vi "Wrapper Fulfill Future.vi"(8 "error in (no error)":errorcluster, 10 "Variant":variant, 11 "Promise in":refnum<class "Promise.lvclass">) -> (0 "error out":errorcluster)   [LabVIEW 2017, in "Promise Future.lvlib" / "Promise.lvclass"]
uses:
  Promise.lvclass
  Promise.lvclass/Promise.ctl
  Future/Future.lvclass
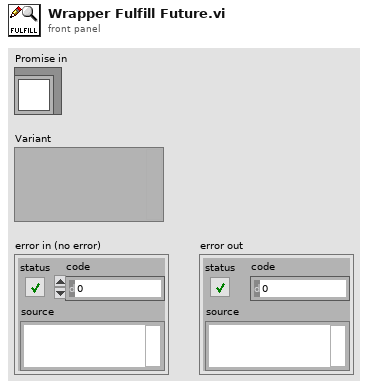
[diagram p1: front panel]
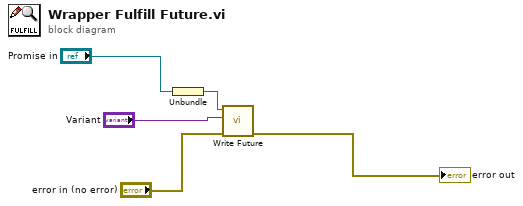
[diagram p0: block diagram]
diagram:
  n1 = Unbundle("Promise in") -> (w1:refnum<class "Future.lvclass">)
  n2 = call "Write Future.vi"("error in (no error)"="error in (no error)", "Value"="Variant", "Future in"=w1) -> ("error out"=→"error out":errorcluster)  [unwired: 7 in, 1 out]
